vi "qiyi.vi"() -> ()   [LabVIEW 2021]
doc: "This samples demonstrates how to sample continuous waveform."
uses:
  <vilib>/Instr/_visa.llb/VISA Configure Serial Port (Instr).vi
  <userlib>/ArtScope/Fetch/ArtScope_FetchVoltage.vi
panel:
  in  "?":enum32{"View", "control", "log"}(tab)
  out "?":bool
  out "波形图":dbl[][](graph)
  in  "退出程序":bool
  in  "TriggerSource":string(combo)="VAL_TRIGGER_CH0"
  in  "TriggerLevel(mV)":sgl
  in  "TriggerWindow(ns)":i32
  in  "TriggerSlope":i32(ring) items=["Negative", "Positive", "NegatPosit"]
  in  "Resource Name":string="Dev1"
  in  "Channel Name":string="0,1"
  in  "Timeout(s)":dbl=10.0
  in  "Vertical Range(V)":i32(ring) items=["-5-+5V", "-1-+1V"]
  in  "Coupling":i32(ring) items=["DC", "AC"]
  in  "MinSampleRate":dbl=40000000.0
  in  "MinRecordLength":i32=100000
  in  "波特率":u64(ring) items=["9600"=9600, "14400"=14400, "115200"=115200]
  out "serial_state":bool
  in  "serial":refnum<visa-resource-name> caption="串口名称"
  in  "打开串口":bool
  in  "写出数据":string
  in  "send":bool
  in  "开始运行":bool
  in  "纳秒脉冲周期":u32
  in  "纳秒脉冲脉宽":u32
  in  "纳秒脉冲个数":i32
  in  "尾切开关参数设置":bool
  in  "微秒脉冲周期":u32
  in  "微秒脉冲脉宽":u32
  in  "微秒脉冲个数":u32
  in  "主开关参数设置":bool
  in  "微秒脉冲延时":u32
  in  "参数下发":bool
  in  "降压放电":bool
  in  "停止设备":bool
  out "读入数据":string
  out "ErrorOutput":errorcluster
  # "Vertical"
  # "Horizontal"
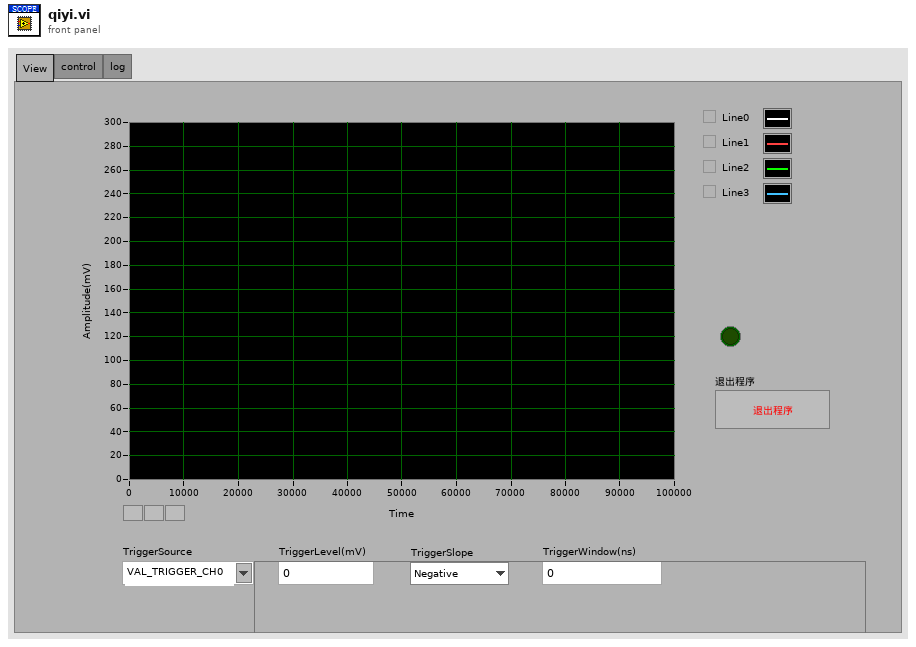
[diagram p1: front panel]
types:
  T1 = typedef "状态机.ctl" = enum16{"Init", "Wait", "GetData", "Exit"}
  T2 = typedef "发送数据处理控件.ctl" = enum16{"0", "1", "2", "3", "4", "5", "6", "7", "8", "9", "exit"}
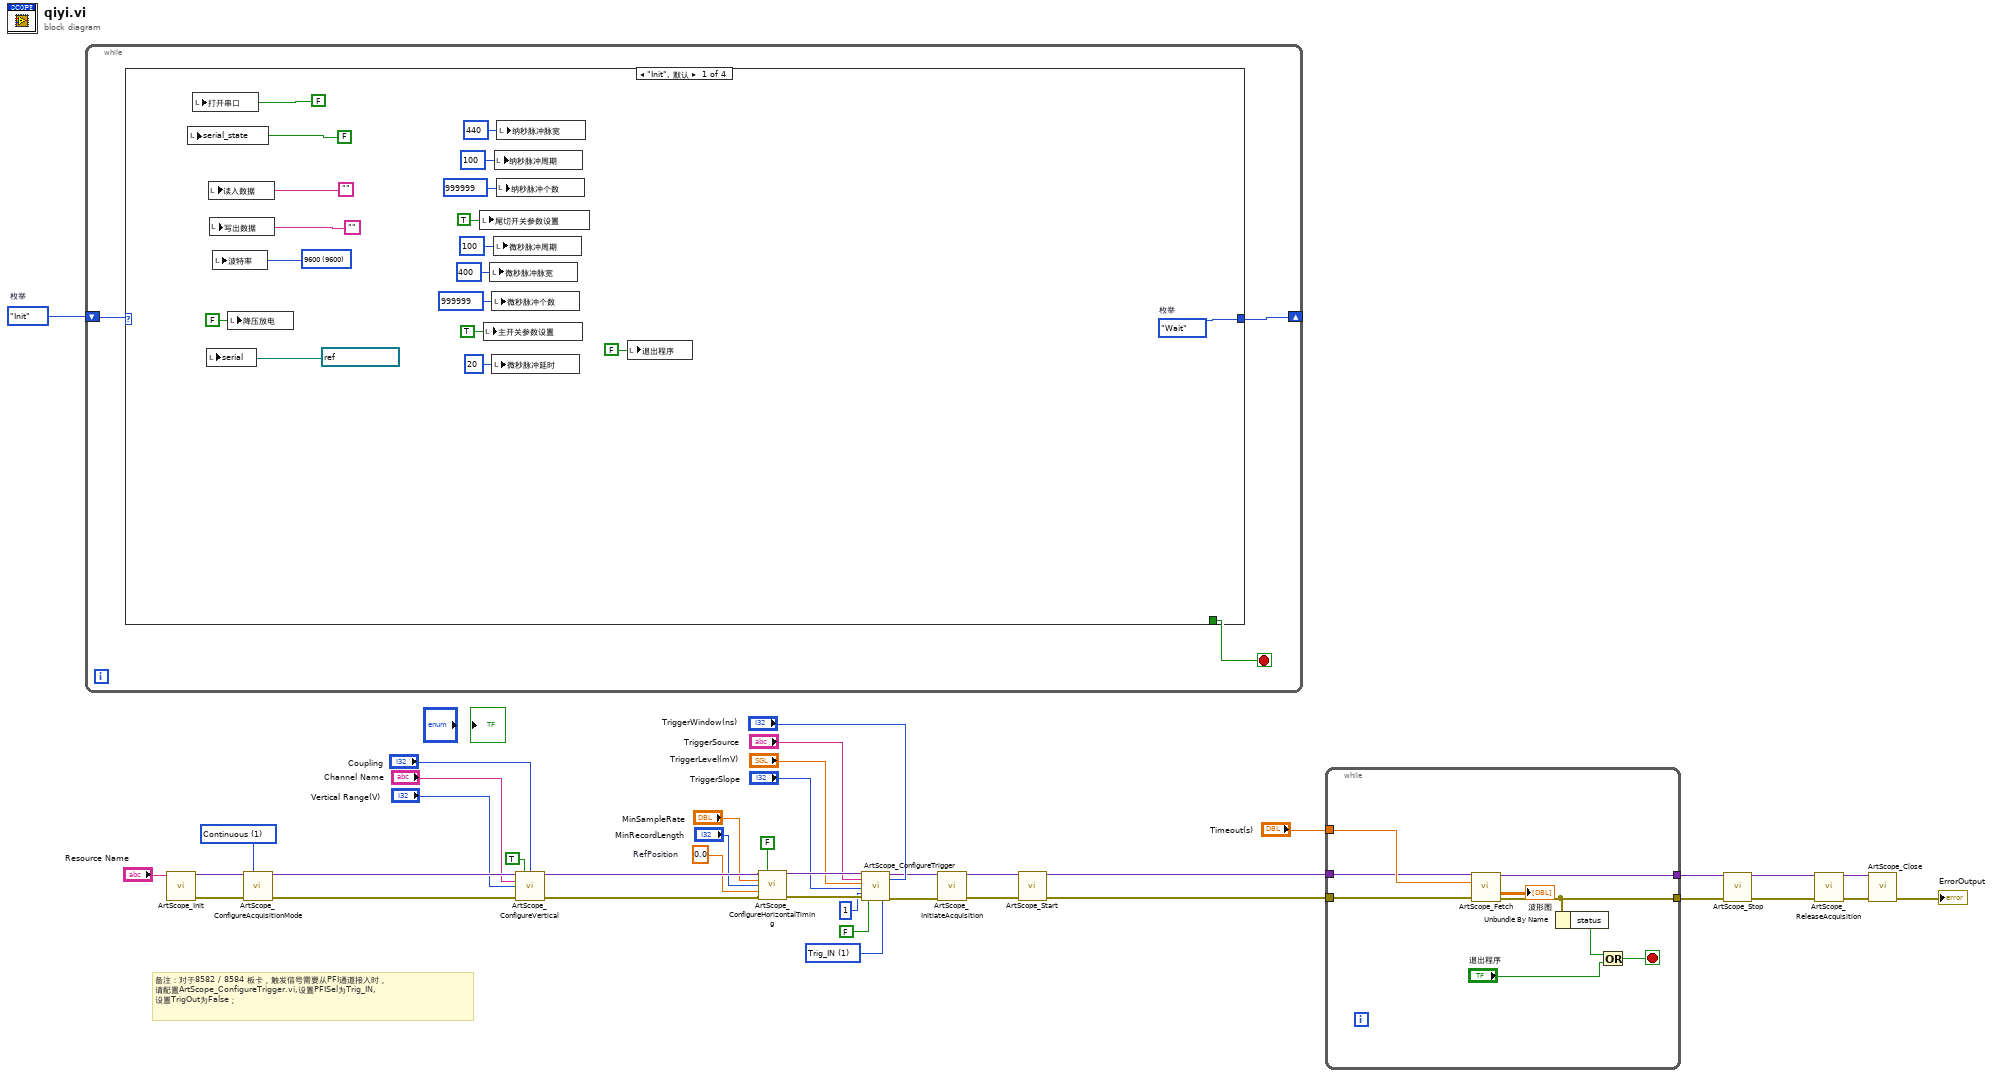
[diagram p0: block diagram]
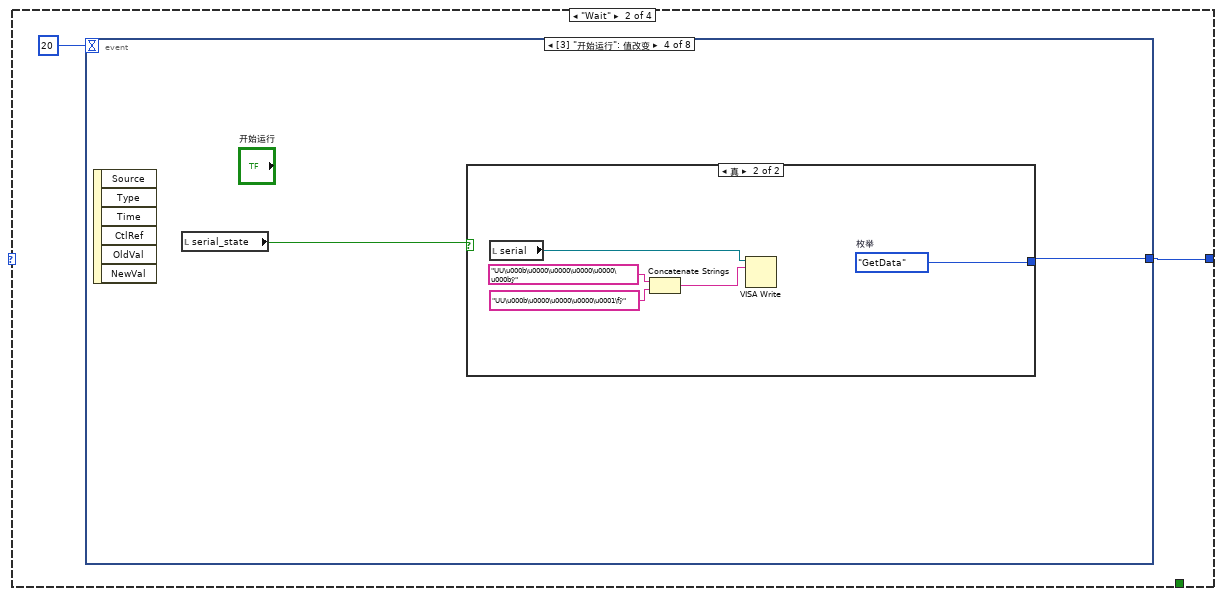
[diagram p2: hidden frame]
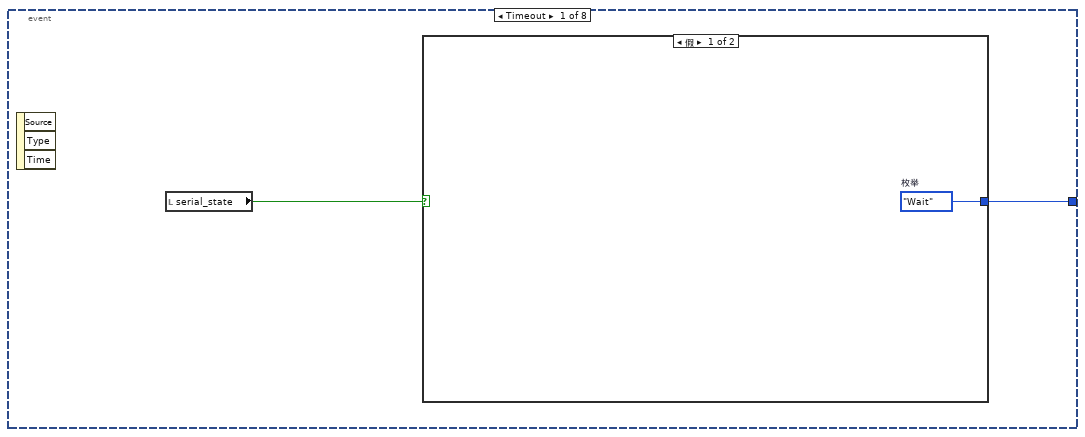
[diagram p3: hidden frame]
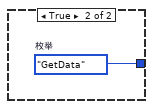
[diagram p4: hidden frame]
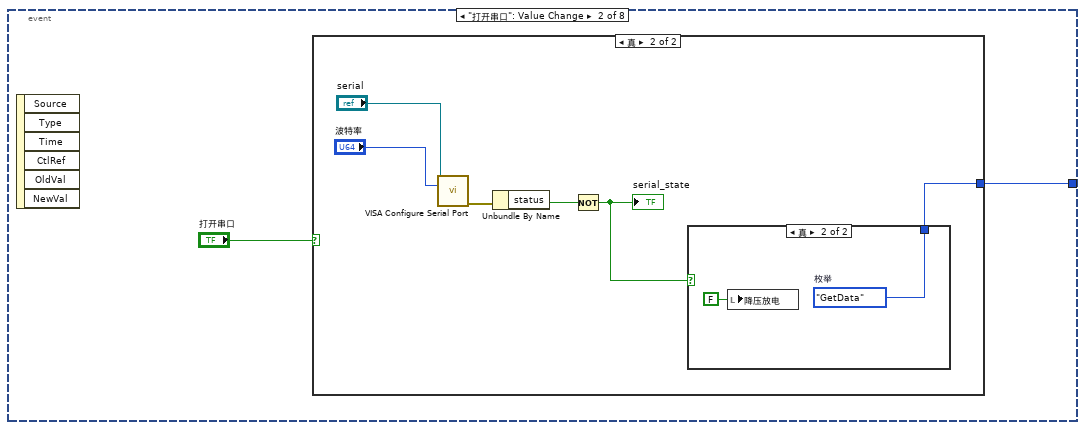
[diagram p5: hidden frame]
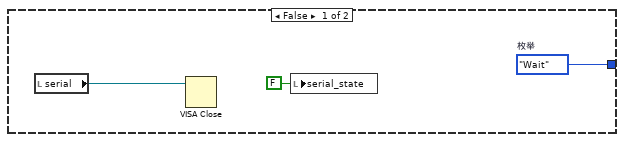
[diagram p6: hidden frame]
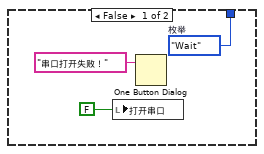
[diagram p7: hidden frame]
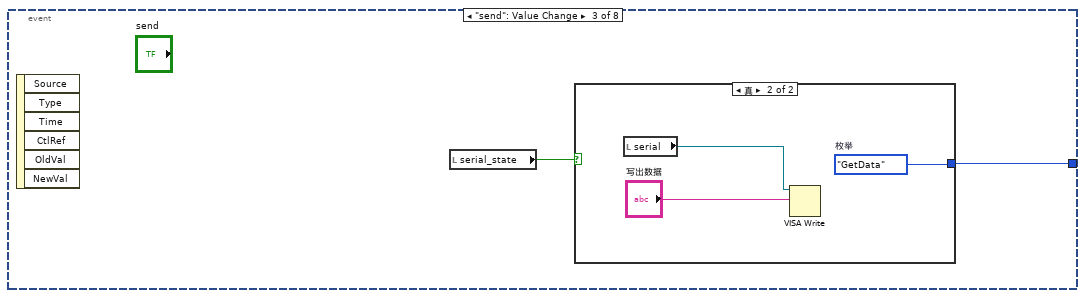
[diagram p8: hidden frame]
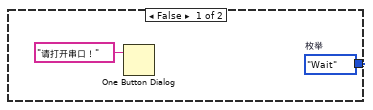
[diagram p9: hidden frame]
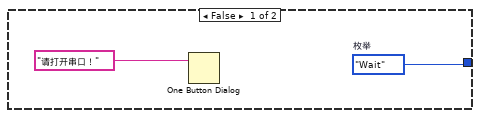
[diagram p10: hidden frame]
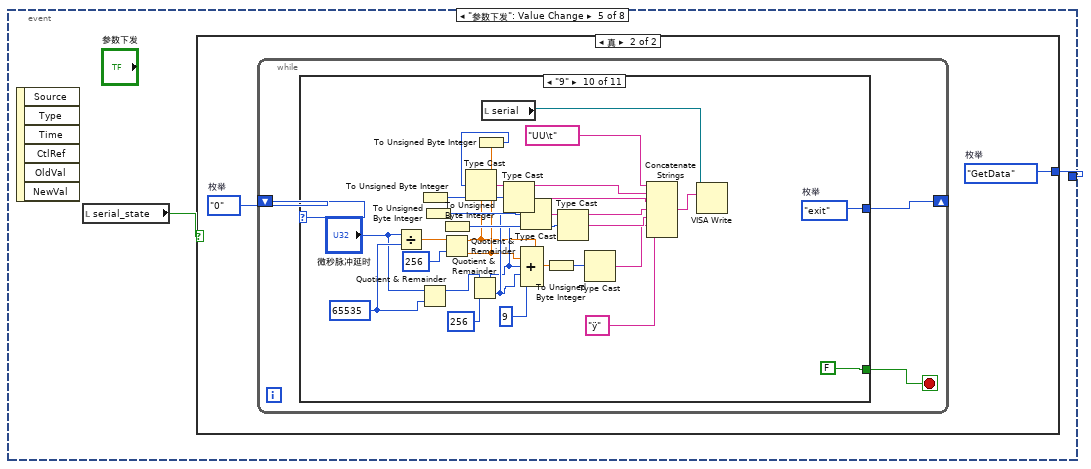
[diagram p11: hidden frame]
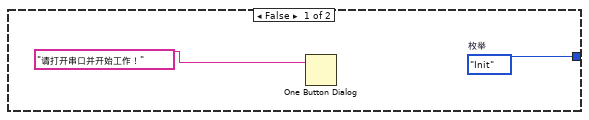
[diagram p12: hidden frame]
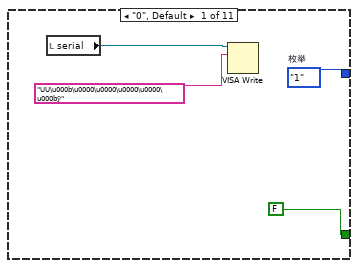
[diagram p13: hidden frame]
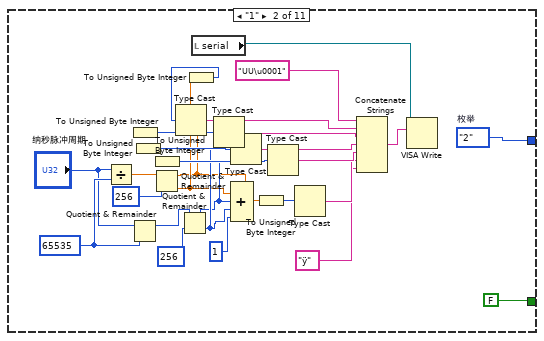
[diagram p14: hidden frame]
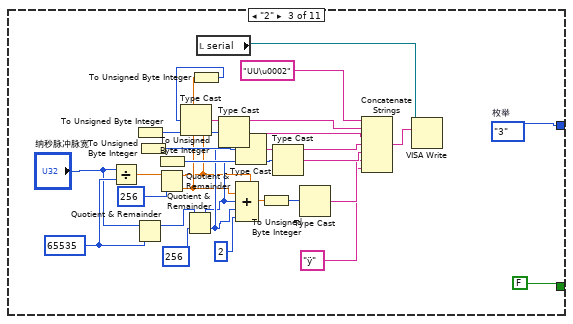
[diagram p15: hidden frame]
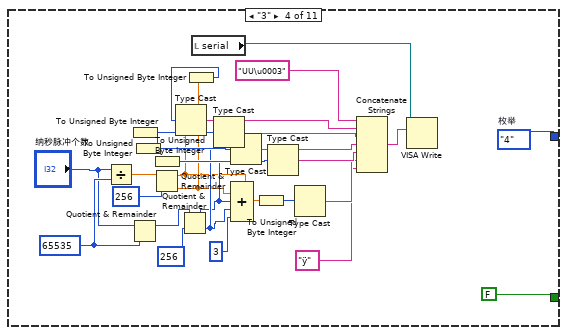
[diagram p16: hidden frame]
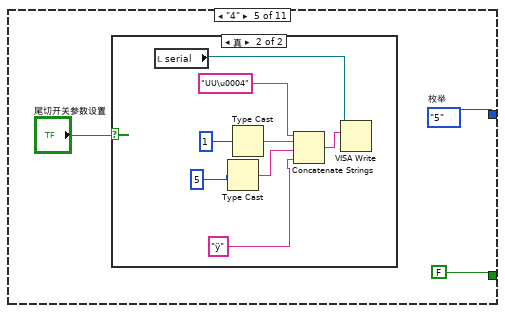
[diagram p17: hidden frame]
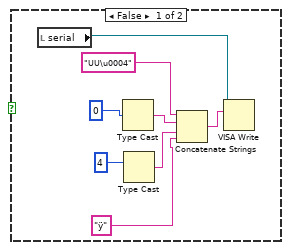
[diagram p18: hidden frame]
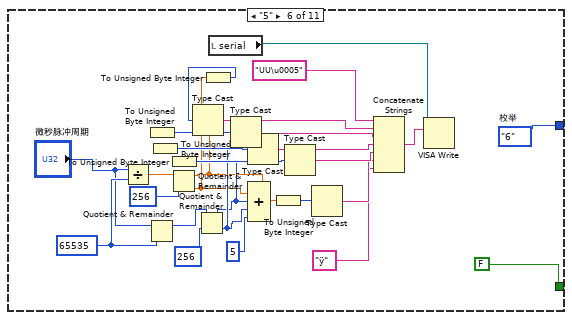
[diagram p19: hidden frame]
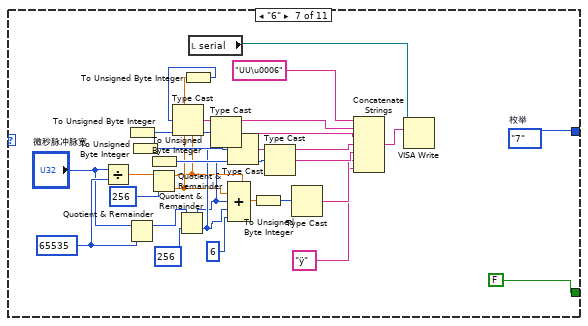
[diagram p20: hidden frame]
diagram:
  w4 = 1 items=["Trig_OUT", "Trig_IN"] ("PFISel")
  w22 = 0.0  # RefPosition
  w36 = 1 items=["Finite", "Continuous"] ("AcuqMode")
  w40 = 状态机."Init"  # 枚举
  # "备注：对于8582 / 8584 板卡，触发信号需要从PFI通道接入时，\n请配置ArtScope_ConfigureTrigger.vi,设置PFISel为Trig_IN,\n设置TrigOut为False；"
  n1 = while {
    shift-right: [w42] -> _
    shift-left: w40 -> [w43]
    stop <- w41 stop-if-true
    n2 = case shown="\"Init\", 默认" w43 {
      tunnel: [w59 w62 w380 w397] -> w42
      tunnel: [_ _ _ TRUE] -> w41
      frame "Init", Default {
        w56 = u64 9600 items=["9600"=9600, "115200"=115200] ("baud rate")
        w59 = 状态机."Wait"  # 枚举
        n3 = local write "serial_state"(FALSE ("serial_state")) -> ()
        n4 = local write "打开串口"(FALSE ("serial_open")) -> ()
        n5 = local write "serial"(refnum<visa-resource-name> "COM6" ("serial")) -> ()
        n6 = local write "读入数据"("") -> ()
        n7 = local write "写出数据"("") -> ()
        n8 = local write "波特率"(w56) -> ()
        n9 = local write "降压放电"(FALSE ("降压放电")) -> ()
        n10 = local write "尾切开关参数设置"(TRUE ("尾切开关参数设置")) -> ()
        n11 = local write "主开关参数设置"(TRUE ("主开关参数设置")) -> ()
        n12 = local write "微秒脉冲脉宽"(u32 400 ("微秒脉冲脉宽")) -> ()
        n13 = local write "微秒脉冲个数"(u32 999999 ("微秒脉冲个数")) -> ()
        n14 = local write "微秒脉冲延时"(u32 20 ("微秒脉冲延时")) -> ()
        n15 = local write "微秒脉冲周期"(u32 100 ("微秒脉冲周期")) -> ()
        n16 = local write "纳秒脉冲周期"(u32 100 ("纳秒脉冲周期")) -> ()
        n17 = local write "纳秒脉冲个数"(999999 ("纳秒脉冲个数")) -> ()
        n18 = local write "纳秒脉冲脉宽"(u32 440 ("纳秒脉冲脉宽")) -> ()
        n19 = local write "退出程序"(FALSE ("退出程序")) -> ()
      }
      frame "Wait" {
        n20 = event shown="[3] \"开始运行\": 值改变" {
          selector: _ -> [_ _ _ _ _ _ _ _]
          dyn-events: _ -> [_ _ _ _ _ _ _ _]
          timeout: 20 -> [_ _ _ _ _ _ _ _]
          tunnel: [w64 w68 w84 w91 w101 w350 w369 w379] -> w62
          event Timeout {
            n21 = event-data() -> ()  [unwired: 1 in, 3 out]
            n22 = local read "serial_state"() -> (w65:bool)
            n23 = case shown="假" w65 {
              tunnel: [w66 w67] -> w64
              frame False {
                w66 = 状态机."Wait"  # 枚举
              }
              frame True {
                w67 = 状态机."GetData"  # 枚举
              }
            }
          }
          event "打开串口": Value Change {
            n24 = event-data() -> ()  [unwired: 1 in, 6 out]
            n25 = case shown="真" "打开串口" {
              tunnel: [w70 w74] -> w68
              frame False {
                w70 = 状态机."Wait"  # 枚举
                n26 = local read "serial"() -> (w72:refnum<visa-resource-name>)
                n27 = VISA Close(VISA resource name=w72) -> ()  [unwired: 1 in, 1 out]
                n28 = local write "serial_state"(FALSE ("serial_state")) -> ()
              }
              frame True {
                n29 = call-poly "VISA Configure Serial Port"("VISA resource name"="serial", "baud rate (9600)"="波特率") -> ("error out"=w77:errorcluster)  [unwired: 12 in, 1 out]
                n30 = Unbundle By Name(w77) -> ("status"=w76:bool)
                n31 = Not(x=w76) -> (.not. x?=w75:bool)
                "serial_state" <- w75
                n32 = case shown="真" w75 {
                  tunnel: [w79 w83] -> w74
                  frame False {
                    w79 = 状态机."Wait"  # 枚举
                    n33 = local write "打开串口"(FALSE ("serial_open")) -> ()
                    n34 = One Button Dialog(message="串口打开失败！" ("消息")) -> ()  [unwired: 1 in, 1 out]
                  }
                  frame True {
                    w83 = 状态机."GetData"  # 枚举
                    n35 = local write "降压放电"(FALSE ("降压放电")) -> ()
                  }
                }
              }
            }
          }
          event "send": Value Change {
            n36 = event-data() -> ()  [unwired: 1 in, 6 out]
            n37 = local read "serial_state"() -> (w85:bool)
            n38 = case shown="真" w85 {
              tunnel: [w86 w88] -> w84
              frame False {
                w86 = 状态机."Wait"  # 枚举
                n39 = One Button Dialog(message="请打开串口！" ("消息")) -> ()  [unwired: 1 in, 1 out]
              }
              frame True {
                w88 = 状态机."GetData"  # 枚举
                n40 = local read "serial"() -> (w89:refnum<visa-resource-name>)
                n41 = VISA Write(VISA resource name=w89, write buffer="写出数据") -> ()  [unwired: 1 in, 3 out]
              }
            }
          }
          event "开始运行": Value Change {
            n42 = event-data() -> ()  [unwired: 1 in, 6 out]
            n43 = local read "serial_state"() -> (w92:bool)
            n44 = case shown="真" w92 {
              tunnel: [w93 w99] -> w91
              frame False {
                w93 = 状态机."Wait"  # 枚举
                n45 = One Button Dialog(message="请打开串口！" ("消息")) -> ()  [unwired: 1 in, 1 out]
              }
              frame True {
                w99 = 状态机."GetData"  # 枚举
                n46 = local read "serial"() -> (w98:refnum<visa-resource-name>)
                n47 = Concatenate Strings("UU\u000b\u0000\u0000\u0000\u0000\u000bÿ" ("写入缓冲区"), "UU\u000b\u0000\u0000\u0000\u0001\fÿ") -> (w95:string)
                n48 = VISA Write(VISA resource name=w98, write buffer=w95) -> ()  [unwired: 1 in, 3 out]
              }
            }
          }
          event "参数下发": Value Change {
            n49 = event-data() -> ()  [unwired: 1 in, 6 out]
            n50 = local read "serial_state"() -> (w100:bool)
            n51 = case shown="真" w100 {
              tunnel: [w102 w105] -> w101
              frame False {
                w102 = 状态机."Init"  # 枚举
                n52 = One Button Dialog(message="请打开串口并开始工作！" ("消息")) -> ()  [unwired: 1 in, 1 out]
              }
              frame True {
                w104 = 发送数据处理控件."0"  # 枚举
                w105 = 状态机."GetData"  # 枚举
                n53 = while {
                  shift-right: [w107] -> _
                  shift-left: w104 -> [w108]
                  stop <- w106 stop-if-true
                  n54 = case shown="\"9\"" w108 {
                    tunnel: [w110 w139 w168 w196 w199 w243 w271 w299 w302 w346 w347] -> w107
                    tunnel: [FALSE FALSE FALSE FALSE FALSE FALSE FALSE FALSE FALSE FALSE TRUE] -> w106
                    frame "0", Default {
                      w110 = 发送数据处理控件."1"  # 枚举
                      n55 = local read "serial"() -> (w112:refnum<visa-resource-name>)
                      n56 = VISA Write(VISA resource name=w112, write buffer="UU\u000b\u0000\u0000\u0000\u0000\u000bÿ" ("写入缓冲区")) -> ()  [unwired: 1 in, 3 out]
                    }
                    frame "1" {
                      w131 = u32 65535 ("y")
                      w139 = 发送数据处理控件."2"  # 枚举
                      n57 = Divide(x="纳秒脉冲周期", y=w131) -> (x/y=w130:dbl)
                      n58 = Quotient & Remainder(x="纳秒脉冲周期", y=w131) -> (x-y*floor(x/y)=w127:u32)  [unwired: 1 out]
                      n59 = Quotient & Remainder(x=w130, y=u32 256) -> (x-y*floor(x/y)=w113:dbl, floor(x/y)=w114:dbl)
                      n60 = To Unsigned Byte Integer(number=w113) -> (unsigned 8bit integer=w124:u8)
                      n61 = Quotient & Remainder(x=w127, y=u32 256) -> (x-y*floor(x/y)=w117:u32, floor(x/y)=w118:u32)
                      n62 = To Unsigned Byte Integer(number=w118) -> (unsigned 8bit integer=w123:u8)
                      n63 = To Unsigned Byte Integer(number=w117) -> (unsigned 8bit integer=w122:u8)
                      n64 = To Unsigned Byte Integer(number=w114) -> (unsigned 8bit integer=w125:u8)
                      n65 = Type Cast(x=w125) -> (*(type *) &x=w132:string)  [unwired: 1 in]
                      n66 = local read "serial"() -> (w140:refnum<visa-resource-name>)
                      n67 = Type Cast(x=w124) -> (*(type *) &x=w121:string)  [unwired: 1 in]
                      n68 = Type Cast(x=w123) -> (*(type *) &x=w120:string)  [unwired: 1 in]
                      n69 = Compound Arithmetic op=ADD(w113, w114, w117, w118, u32 1 ("值")) -> (w128:dbl)
                      n70 = To Unsigned Byte Integer(number=w128) -> (unsigned 8bit integer=w129:u8)
                      n71 = Type Cast(x=w122) -> (*(type *) &x=w119:string)  [unwired: 1 in]
                      n72 = Type Cast(x=w129) -> (*(type *) &x=w116:string)  [unwired: 1 in]
                      n73 = Concatenate Strings("UU\u0001" ("写入缓冲区"), w132, w121, w120, w119, w116, "ÿ") -> (w137:string)
                      n74 = VISA Write(VISA resource name=w140, write buffer=w137) -> ()  [unwired: 1 in, 3 out]
                    }
                    frame "2" {
                      w159 = u32 65535 ("y")
                      w168 = 发送数据处理控件."3"  # 枚举
                      n75 = Divide(x="纳秒脉冲脉宽", y=w159) -> (x/y=w158:dbl)
                      n76 = Quotient & Remainder(x="纳秒脉冲脉宽", y=w159) -> (x-y*floor(x/y)=w155:u32)  [unwired: 1 out]
                      n77 = Quotient & Remainder(x=w158, y=u32 256) -> (x-y*floor(x/y)=w141:dbl, floor(x/y)=w142:dbl)
                      n78 = To Unsigned Byte Integer(number=w141) -> (unsigned 8bit integer=w153:u8)
                      n79 = Quotient & Remainder(x=w155, y=u32 256) -> (x-y*floor(x/y)=w146:u32, floor(x/y)=w147:u32)
                      n80 = To Unsigned Byte Integer(number=w147) -> (unsigned 8bit integer=w152:u8)
                      n81 = To Unsigned Byte Integer(number=w146) -> (unsigned 8bit integer=w151:u8)
                      n82 = To Unsigned Byte Integer(number=w142) -> (unsigned 8bit integer=w154:u8)
                      n83 = Type Cast(x=w154) -> (*(type *) &x=w160:string)  [unwired: 1 in]
                      n84 = local read "serial"() -> (w166:refnum<visa-resource-name>)
                      n85 = Type Cast(x=w153) -> (*(type *) &x=w150:string)  [unwired: 1 in]
                      n86 = Type Cast(x=w152) -> (*(type *) &x=w149:string)  [unwired: 1 in]
                      n87 = Compound Arithmetic op=ADD(w141, w142, w146, w147, u32 2 ("值")) -> (w156:dbl)
                      n88 = To Unsigned Byte Integer(number=w156) -> (unsigned 8bit integer=w157:u8)
                      n89 = Type Cast(x=w151) -> (*(type *) &x=w148:string)  [unwired: 1 in]
                      n90 = Type Cast(x=w157) -> (*(type *) &x=w145:string)  [unwired: 1 in]
                      n91 = Concatenate Strings("UU\u0002" ("写入缓冲区"), w160, w150, w149, w148, w145, "ÿ") -> (w164:string)
                      n92 = VISA Write(VISA resource name=w166, write buffer=w164) -> ()  [unwired: 1 in, 3 out]
                    }
                    frame "3" {
                      w187 = u32 65535 ("y")
                      w196 = 发送数据处理控件."4"  # 枚举
                      n93 = Divide(x="纳秒脉冲个数", y=w187) -> (x/y=w186:dbl)
                      n94 = Quotient & Remainder(x="纳秒脉冲个数", y=w187) -> (x-y*floor(x/y)=w183:u32)  [unwired: 1 out]
                      n95 = Quotient & Remainder(x=w186, y=u32 256) -> (x-y*floor(x/y)=w169:dbl, floor(x/y)=w170:dbl)
                      n96 = To Unsigned Byte Integer(number=w169) -> (unsigned 8bit integer=w181:u8)
                      n97 = Quotient & Remainder(x=w183, y=u32 256) -> (x-y*floor(x/y)=w174:u32, floor(x/y)=w175:u32)
                      n98 = To Unsigned Byte Integer(number=w175) -> (unsigned 8bit integer=w180:u8)
                      n99 = To Unsigned Byte Integer(number=w174) -> (unsigned 8bit integer=w179:u8)
                      n100 = To Unsigned Byte Integer(number=w170) -> (unsigned 8bit integer=w182:u8)
                      n101 = Type Cast(x=w182) -> (*(type *) &x=w188:string)  [unwired: 1 in]
                      n102 = local read "serial"() -> (w194:refnum<visa-resource-name>)
                      n103 = Type Cast(x=w181) -> (*(type *) &x=w178:string)  [unwired: 1 in]
                      n104 = Type Cast(x=w180) -> (*(type *) &x=w177:string)  [unwired: 1 in]
                      n105 = Compound Arithmetic op=ADD(w169, w170, w174, w175, u32 3 ("值")) -> (w184:dbl)
                      n106 = To Unsigned Byte Integer(number=w184) -> (unsigned 8bit integer=w185:u8)
                      n107 = Type Cast(x=w179) -> (*(type *) &x=w176:string)  [unwired: 1 in]
                      n108 = Type Cast(x=w185) -> (*(type *) &x=w173:string)  [unwired: 1 in]
                      n109 = Concatenate Strings("UU\u0003" ("写入缓冲区"), w188, w178, w177, w176, w173, "ÿ") -> (w192:string)
                      n110 = VISA Write(VISA resource name=w194, write buffer=w192) -> ()  [unwired: 1 in, 3 out]
                    }
                    frame "4" {
                      w199 = 发送数据处理控件."5"  # 枚举
                      n111 = case shown="真" "尾切开关参数设置" {
                        frame False {
                          n112 = local read "serial"() -> (w207:refnum<visa-resource-name>)
                          n113 = Type Cast(x=u32 0 ("数字")) -> (*(type *) &x=w202:string)  [unwired: 1 in]
                          n114 = Type Cast(x=u8 4 ("宽度(-)")) -> (*(type *) &x=w200:string)  [unwired: 1 in]
                          n115 = Concatenate Strings("UU\u0004" ("写入缓冲区"), w202, w200, "ÿ") -> (w206:string)
                          n116 = VISA Write(VISA resource name=w207, write buffer=w206) -> ()  [unwired: 1 in, 3 out]
                        }
                        frame True {
                          n117 = local read "serial"() -> (w215:refnum<visa-resource-name>)
                          n118 = Type Cast(x=u8 5 ("宽度(-)")) -> (*(type *) &x=w208:string)  [unwired: 1 in]
                          n119 = Type Cast(x=u32 1 ("数字")) -> (*(type *) &x=w210:string)  [unwired: 1 in]
                          n120 = Concatenate Strings("UU\u0004" ("写入缓冲区"), w210, w208, "ÿ") -> (w214:string)
                          n121 = VISA Write(VISA resource name=w215, write buffer=w214) -> ()  [unwired: 1 in, 3 out]
                        }
                      }
                    }
                    frame "5" {
                      w234 = u32 65535 ("y")
                      w243 = 发送数据处理控件."6"  # 枚举
                      n122 = Divide(x="微秒脉冲周期", y=w234) -> (x/y=w233:dbl)
                      n123 = Quotient & Remainder(x="微秒脉冲周期", y=w234) -> (x-y*floor(x/y)=w230:u32)  [unwired: 1 out]
                      n124 = Quotient & Remainder(x=w233, y=u32 256) -> (x-y*floor(x/y)=w216:dbl, floor(x/y)=w217:dbl)
                      n125 = To Unsigned Byte Integer(number=w216) -> (unsigned 8bit integer=w228:u8)
                      n126 = Quotient & Remainder(x=w230, y=u32 256) -> (x-y*floor(x/y)=w221:u32, floor(x/y)=w222:u32)
                      n127 = To Unsigned Byte Integer(number=w222) -> (unsigned 8bit integer=w227:u8)
                      n128 = To Unsigned Byte Integer(number=w221) -> (unsigned 8bit integer=w226:u8)
                      n129 = To Unsigned Byte Integer(number=w217) -> (unsigned 8bit integer=w229:u8)
                      n130 = Type Cast(x=w229) -> (*(type *) &x=w235:string)  [unwired: 1 in]
                      n131 = local read "serial"() -> (w241:refnum<visa-resource-name>)
                      n132 = Type Cast(x=w228) -> (*(type *) &x=w225:string)  [unwired: 1 in]
                      n133 = Type Cast(x=w227) -> (*(type *) &x=w224:string)  [unwired: 1 in]
                      n134 = Compound Arithmetic op=ADD(w216, w217, w221, w222, u32 5 ("值")) -> (w231:dbl)
                      n135 = To Unsigned Byte Integer(number=w231) -> (unsigned 8bit integer=w232:u8)
                      n136 = Type Cast(x=w226) -> (*(type *) &x=w223:string)  [unwired: 1 in]
                      n137 = Type Cast(x=w232) -> (*(type *) &x=w220:string)  [unwired: 1 in]
                      n138 = Concatenate Strings("UU\u0005" ("写入缓冲区"), w235, w225, w224, w223, w220, "ÿ") -> (w239:string)
                      n139 = VISA Write(VISA resource name=w241, write buffer=w239) -> ()  [unwired: 1 in, 3 out]
                    }
                    frame "6" {
                      w262 = u32 65535 ("y")
                      w271 = 发送数据处理控件."7"  # 枚举
                      n140 = Divide(x="微秒脉冲脉宽", y=w262) -> (x/y=w261:dbl)
                      n141 = Quotient & Remainder(x="微秒脉冲脉宽", y=w262) -> (x-y*floor(x/y)=w258:u32)  [unwired: 1 out]
                      n142 = Quotient & Remainder(x=w261, y=u32 256) -> (x-y*floor(x/y)=w244:dbl, floor(x/y)=w245:dbl)
                      n143 = To Unsigned Byte Integer(number=w244) -> (unsigned 8bit integer=w256:u8)
                      n144 = Quotient & Remainder(x=w258, y=u32 256) -> (x-y*floor(x/y)=w249:u32, floor(x/y)=w250:u32)
                      n145 = To Unsigned Byte Integer(number=w250) -> (unsigned 8bit integer=w255:u8)
                      n146 = To Unsigned Byte Integer(number=w249) -> (unsigned 8bit integer=w254:u8)
                      n147 = To Unsigned Byte Integer(number=w245) -> (unsigned 8bit integer=w257:u8)
                      n148 = Type Cast(x=w257) -> (*(type *) &x=w263:string)  [unwired: 1 in]
                      n149 = local read "serial"() -> (w269:refnum<visa-resource-name>)
                      n150 = Type Cast(x=w256) -> (*(type *) &x=w253:string)  [unwired: 1 in]
                      n151 = Type Cast(x=w255) -> (*(type *) &x=w252:string)  [unwired: 1 in]
                      n152 = Compound Arithmetic op=ADD(w244, w245, w249, w250, u32 6 ("值")) -> (w259:dbl)
                      n153 = To Unsigned Byte Integer(number=w259) -> (unsigned 8bit integer=w260:u8)
                      n154 = Type Cast(x=w254) -> (*(type *) &x=w251:string)  [unwired: 1 in]
                      n155 = Type Cast(x=w260) -> (*(type *) &x=w248:string)  [unwired: 1 in]
                      n156 = Concatenate Strings("UU\u0006" ("写入缓冲区"), w263, w253, w252, w251, w248, "ÿ") -> (w267:string)
                      n157 = VISA Write(VISA resource name=w269, write buffer=w267) -> ()  [unwired: 1 in, 3 out]
                    }
                    frame "7" {
                      w290 = u32 65535 ("y")
                      w299 = 发送数据处理控件."8"  # 枚举
                      n158 = Divide(x="微秒脉冲个数", y=w290) -> (x/y=w289:dbl)
                      n159 = Quotient & Remainder(x="微秒脉冲个数", y=w290) -> (x-y*floor(x/y)=w286:u32)  [unwired: 1 out]
                      n160 = Quotient & Remainder(x=w289, y=u32 256) -> (x-y*floor(x/y)=w272:dbl, floor(x/y)=w273:dbl)
                      n161 = To Unsigned Byte Integer(number=w272) -> (unsigned 8bit integer=w284:u8)
                      n162 = Quotient & Remainder(x=w286, y=u32 256) -> (x-y*floor(x/y)=w277:u32, floor(x/y)=w278:u32)
                      n163 = To Unsigned Byte Integer(number=w278) -> (unsigned 8bit integer=w283:u8)
                      n164 = To Unsigned Byte Integer(number=w277) -> (unsigned 8bit integer=w282:u8)
                      n165 = To Unsigned Byte Integer(number=w273) -> (unsigned 8bit integer=w285:u8)
                      n166 = Type Cast(x=w285) -> (*(type *) &x=w291:string)  [unwired: 1 in]
                      n167 = local read "serial"() -> (w297:refnum<visa-resource-name>)
                      n168 = Type Cast(x=w284) -> (*(type *) &x=w281:string)  [unwired: 1 in]
                      n169 = Type Cast(x=w283) -> (*(type *) &x=w280:string)  [unwired: 1 in]
                      n170 = Compound Arithmetic op=ADD(w272, w273, w277, w278, u32 7 ("值")) -> (w287:dbl)
                      n171 = To Unsigned Byte Integer(number=w287) -> (unsigned 8bit integer=w288:u8)
                      n172 = Type Cast(x=w282) -> (*(type *) &x=w279:string)  [unwired: 1 in]
                      n173 = Type Cast(x=w288) -> (*(type *) &x=w276:string)  [unwired: 1 in]
                      n174 = Concatenate Strings("UU\u0007" ("写入缓冲区"), w291, w281, w280, w279, w276, "ÿ") -> (w295:string)
                      n175 = VISA Write(VISA resource name=w297, write buffer=w295) -> ()  [unwired: 1 in, 3 out]
                    }
                    frame "8" {
                      w302 = 发送数据处理控件."9"  # 枚举
                      n176 = case shown="假" "主开关参数设置" {
                        frame False {
                          n177 = local read "serial"() -> (w310:refnum<visa-resource-name>)
                          n178 = Type Cast(x=u32 0 ("数字")) -> (*(type *) &x=w305:string)  [unwired: 1 in]
                          n179 = Type Cast(x=u8 8 ("宽度(-)")) -> (*(type *) &x=w303:string)  [unwired: 1 in]
                          n180 = Concatenate Strings("UU\b" ("写入缓冲区"), w305, w303, "ÿ") -> (w309:string)
                          n181 = VISA Write(VISA resource name=w310, write buffer=w309) -> ()  [unwired: 1 in, 3 out]
                        }
                        frame True {
                          n182 = local read "serial"() -> (w318:refnum<visa-resource-name>)
                          n183 = Type Cast(x=u32 1 ("数字")) -> (*(type *) &x=w314:string)  [unwired: 1 in]
                          n184 = Type Cast(x=u8 9 ("宽度(-)")) -> (*(type *) &x=w311:string)  [unwired: 1 in]
                          n185 = Concatenate Strings("UU\b" ("写入缓冲区"), w314, w311, "ÿ") -> (w317:string)
                          n186 = VISA Write(VISA resource name=w318, write buffer=w317) -> ()  [unwired: 1 in, 3 out]
                        }
                      }
                    }
                    frame "9" {
                      w326 = u32 65535 ("y")
                      w346 = 发送数据处理控件."exit"  # 枚举
                      n187 = Divide(x="微秒脉冲延时", y=w326) -> (x/y=w341:dbl)
                      n188 = Quotient & Remainder(x="微秒脉冲延时", y=w326) -> (x-y*floor(x/y)=w338:u32)  [unwired: 1 out]
                      n189 = Quotient & Remainder(x=w341, y=u32 256) -> (x-y*floor(x/y)=w319:dbl, floor(x/y)=w320:dbl)
                      n190 = To Unsigned Byte Integer(number=w319) -> (unsigned 8bit integer=w336:u8)
                      n191 = Quotient & Remainder(x=w338, y=u32 256) -> (x-y*floor(x/y)=w329:u32, floor(x/y)=w330:u32)
                      n192 = To Unsigned Byte Integer(number=w330) -> (unsigned 8bit integer=w335:u8)
                      n193 = To Unsigned Byte Integer(number=w329) -> (unsigned 8bit integer=w334:u8)
                      n194 = To Unsigned Byte Integer(number=w320) -> (unsigned 8bit integer=w337:u8)
                      n195 = Type Cast(x=w337) -> (*(type *) &x=w342:string)  [unwired: 1 in]
                      n196 = local read "serial"() -> (w344:refnum<visa-resource-name>)
                      n197 = Type Cast(x=w336) -> (*(type *) &x=w333:string)  [unwired: 1 in]
                      n198 = Type Cast(x=w335) -> (*(type *) &x=w332:string)  [unwired: 1 in]
                      n199 = Compound Arithmetic op=ADD(w319, w320, w329, w330, u32 9 ("值")) -> (w339:dbl)
                      n200 = To Unsigned Byte Integer(number=w339) -> (unsigned 8bit integer=w340:u8)
                      n201 = Type Cast(x=w334) -> (*(type *) &x=w331:string)  [unwired: 1 in]
                      n202 = Type Cast(x=w340) -> (*(type *) &x=w328:string)  [unwired: 1 in]
                      n203 = Concatenate Strings("UU\t" ("写入缓冲区"), w342, w333, w332, w331, w328, "ÿ") -> (w343:string)
                      n204 = VISA Write(VISA resource name=w344, write buffer=w343) -> ()  [unwired: 1 in, 3 out]
                    }
                    frame "exit" {
                      w347 = 发送数据处理控件."exit"  # 枚举
                    }
                  }
                }
              }
            }
          }
          event "降压放电": Value Change {
            n205 = event-data() -> ()  [unwired: 1 in, 6 out]
            n206 = local read "降压放电"() -> (w349:bool)
            n207 = case shown="假" w349 {
              tunnel: [w351 w361] -> w350
              frame False {
                n208 = local read "serial_state"() -> (w352:bool)
                n209 = case shown="真" w352 {
                  tunnel: [w354 w359] -> w351
                  frame False {
                    w354 = 状态机."Wait"  # 枚举
                    n210 = One Button Dialog(message="请打开串口并开始工作！" ("消息")) -> ()  [unwired: 1 in, 1 out]
                  }
                  frame True {
                    w359 = 状态机."GetData"  # 枚举
                    n211 = local read "serial"() -> (w358:refnum<visa-resource-name>)
                    n212 = Concatenate Strings("UU\u000b\u0000\u0000\u0000\u0000\u000bÿ" ("写入缓冲区"), "UU\n\u0000\u0000\u0000\u0000\nÿ" ("写入缓冲区")) -> (w355:string)
                    n213 = VISA Write(VISA resource name=w358, write buffer=w355) -> ()  [unwired: 1 in, 3 out]
                  }
                }
              }
              frame True {
                n214 = local read "serial_state"() -> (w360:bool)
                n215 = case shown="真" w360 {
                  tunnel: [w363 w368] -> w361
                  frame False {
                    w363 = 状态机."Wait"  # 枚举
                    n216 = One Button Dialog(message="请打开串口并开始工作！" ("消息")) -> ()  [unwired: 1 in, 1 out]
                  }
                  frame True {
                    w368 = 状态机."GetData"  # 枚举
                    n217 = local read "serial"() -> (w367:refnum<visa-resource-name>)
                    n218 = Concatenate Strings("UU\u000b\u0000\u0000\u0000\u0000\u000bÿ" ("写入缓冲区"), "UU\u0004\u0000\u0000\u0000\u0000\u0004ÿ" ("写入缓冲区")) -> (w364:string)
                    n219 = VISA Write(VISA resource name=w367, write buffer=w364) -> ()  [unwired: 1 in, 3 out]
                  }
                }
              }
            }
          }
          event "停止设备": Value Change {
            n220 = event-data() -> ()  [unwired: 1 in, 6 out]
            n221 = local read "serial_state"() -> (w370:bool)
            n222 = case shown="假" w370 {
              tunnel: [w372 w378] -> w369
              frame False {
                w372 = 状态机."Wait"  # 枚举
                n223 = One Button Dialog(message="请打开串口并开始工作！" ("消息")) -> ()  [unwired: 1 in, 1 out]
              }
              frame True {
                w378 = 状态机."GetData"  # 枚举
                n224 = local read "serial"() -> (w377:refnum<visa-resource-name>)
                n225 = Concatenate Strings("UU\u000b\u0000\u0000\u0000\u0000\u000bÿ" ("写入缓冲区"), "UU\u0004\u0000\u0000\u0000\u0000\u0004ÿ" ("写入缓冲区"), "UU\b\u0000\u0000\u0000\u0000\bÿ" ("写入缓冲区")) -> (w374:string)
                n226 = VISA Write(VISA resource name=w377, write buffer=w374) -> ()  [unwired: 1 in, 3 out]
              }
            }
          }
          event "退出程序": Value Change {
            w379 = 状态机."Exit"  # 枚举
            n227 = event-data() -> ()  [unwired: 1 in, 6 out]
          }
        }
      }
      frame "GetData" {
        n228 = local read "serial_state"() -> (w381:bool)
        n229 = case shown="真" w381 {
          tunnel: [w382 w384] -> w380
          frame False {
            w382 = 状态机."Wait"  # 枚举
            n230 = One Button Dialog(message="请打开串口并开始工作！" ("消息")) -> ()  [unwired: 1 in, 1 out]
          }
          frame True {
            w384 = 状态机."Wait"  # 枚举
            n231 = local read "serial"() -> (w385:refnum<visa-resource-name>)
            n232 = property class="Instr"(reference=w385) -> (reference out=w388:refnum<visa-resource-name>, "Serial Settings:Number of Bytes at Serial Port"=w386:u32)  [unwired: 1 in, 1 out]
            n233 = Not Equal To 0?(x=w386) -> (x != 0?=w387:bool)
            n234 = case shown="真" w387 {
              tunnel: w388 -> [_ w394]
              tunnel: w386 -> [_ w393]
              frame False {
              }
              frame True {
                n235 = local read "读入数据"() -> (w390:string)
                n236 = VISA Read(VISA resource name=w394, byte count=w393) -> (read buffer=w391:string)  [unwired: 1 in, 3 out]
                n237 = Concatenate Strings(w390, w391) -> (→"读入数据":string)
                n238 = property on="读入数据" class="Str"("Text.Scroll Position"=inf) -> ()  [unwired: 2 in, 2 out]
              }
            }
          }
        }
      }
      frame "Exit" {
        w397 = 状态机."Exit"  # 枚举
        n239 = local read "serial_state"() -> (w395:bool)
        n240 = case shown="真" w395 {
          frame False {
          }
          frame True {
            n241 = local read "serial"() -> (w400:refnum<visa-resource-name>)
            n242 = local write "serial_state"(FALSE ("serial_state")) -> ()
            n243 = local write "打开串口"(FALSE ("serial_state")) -> ()
            n244 = VISA Close(VISA resource name=w400) -> ()  [unwired: 1 in, 1 out]
          }
        }
      }
    }
  }
  n245 = call <userlib>:"ArtScope_Init.vi"("TaskName"="Resource Name") -> ("TaskHandle"=w39:variant, "ErrorOutput"=w38:errorcluster)  [unwired: 13 in]
  n246 = call <userlib>:"ArtScope_ConfigureAcquisitionMode.vi"("TaskHandle"=w39, "AcquMode"=w36, "ErrorInput"=w38) -> ("TaskHandle"=w35:variant, "ErrorOutput"=w34:errorcluster)  [unwired: 11 in]
  n247 = call <userlib>:"ArtScope_ConfigureVertical.vi"("TaskHandle"=w35, "Enable"=TRUE, "Coupling"="Coupling", "ChannelName"="Channel Name", "Range"="Vertical Range(V)", "ErrorInput"=w34) -> ("TaskHandle"=w31:variant, "ErrorOutput"=w30:errorcluster)  [unwired: 8 in]
  n248 = call <userlib>:"ArtScope_ConfigureHorizontalTiming.vi"("TaskHandle"=w31, "HardwareDelayEnable"=FALSE, "MinSampleRate"="MinSampleRate", "MinNumPts"="MinRecordLength", "RefPosition"=w22, "ErrorInput"=w30) -> ("TaskHandle"=w28:variant, "ErrorOutput"=w27:errorcluster)  [unwired: 8 in]
  n249 = call <userlib>:"ArtScope_ConfigureTrigger.vi"("TaskHandle"=w28, "TriggerSource"="TriggerSource", "TriggerLevel"="TriggerLevel(mV)", "TriggerSlope"="TriggerSlope", "TriggerCount"=1, "ErrorInput"=w27, "TriggerWindow"="TriggerWindow(ns)", "TrigOutEnable"=FALSE, "PFISel"=w4) -> ("TaskHandle"=w15:variant, "ErrorOutput"=w14:errorcluster)  [unwired: 9 in]
  n250 = call <userlib>:"ArtScope_InitiateAcquisition.vi"("TaskHandle"=w15, "ErrorInput"=w14) -> ("TaskHandle"=w12:variant, "ErrorOutput"=w13:errorcluster)  [unwired: 12 in]
  n251 = call <userlib>:"ArtScope_Start.vi"("TaskHandle"=w12, "ErrorInput"=w13) -> ("TaskHandle"=w3:variant, "ErrorOutput"=w2:errorcluster)  [unwired: 12 in]
  n252 = while {
    tunnel: [w409] -> w6
    tunnel: [w406] -> w9
    tunnel: "Timeout(s)" -> [w407]
    tunnel: w3 -> [w403]
    tunnel: w2 -> [w402]
    stop <- w404 stop-if-true
    n253 = call-poly <userlib>:"ArtScope_Fetch.vi"("TaskHandle"=w403, "timeout"=w407, "ErrorInput"=w402) -> ("TaskHandle"=w409:variant, "Data"=→"波形图":dbl[][], "ErrorOutput"=w406:errorcluster)  [unwired: 10 in]
    n254 = Unbundle By Name(w406) -> ("status"=w405:bool)
    n255 = Or(x=w405, y="退出程序") -> (x .or. y?=w404:bool)
  }
  n256 = call <userlib>:"ArtScope_Stop.vi"("TaskHandle"=w6, "ErrorInput"=w9) -> ("TaskHandle"=w7:variant, "ErrorOutput"=w8:errorcluster)  [unwired: 12 in]
  n257 = call <userlib>:"ArtScope_ReleaseAcquisition.vi"("TaskHandle"=w7, "ErrorInput"=w8) -> ("TaskHandle"=w10:variant, "ErrorOutput"=w11:errorcluster)  [unwired: 12 in]
  n258 = call <userlib>:"ArtScope_Close.vi"("TaskHandle"=w10, "ErrorInput"=w11) -> ("ErrorOutput"=→"ErrorOutput":errorcluster)  [unwired: 13 in]
